vi "Build Type Tree.vi"(10 "Value":variant, 11 "Name":string) -> (3 "Type Tree":T1[](array[typedef]))   [LabVIEW 2018, in "LVClassByRef.lvlib"]
uses:
  <resource>/Framework/Providers/LVClassByRef/LVClassByRef.lvlib
  <resource>/Framework/Providers/LVClassByRef/Type Item.ctl
  <resource>/Framework/Providers/LVClassByRef/Tree Item.ctl
  <vilib>/Utility/Data Type/Type Definitions/Data Type.ctl
  <vilib>/Utility/Data Type/NI_Data Type.lvlib
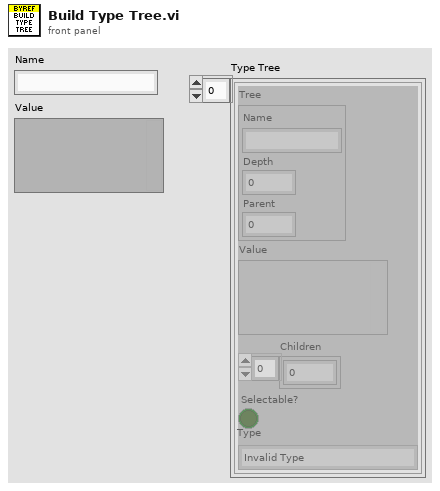
[diagram p1: front panel]
types:
  T1 = typedef "LVClassByRef.lvlib/Type Item.ctl" = cluster{"Tree":T2, "Value":variant, "Children":i32[], "Selectable?":bool, "Type":T3}
  T2 = typedef "LVClassByRef.lvlib/Tree Item.ctl" = cluster{"Name":string, "Depth":i32, "Parent":i32}
  T3 = typedef "NI_Data Type.lvlib/Data Type.ctl" = enum8{"Invalid Type", "Void", "I8", "I16", "I32", "I64", "U8", "U16", "U32", "U64", "Single Float", "Double Float", "Extended Float", "Single Complex", "Double Complex", "Extended Complex", "Enum U8", "Enum U16", "Enum U32", "Enum U64", "Single Float With Unit", "Double Float With Unit", "Extended Float With Unit", "Single Complex with Unit", "Double Complex with Unit", "Extended Complex with Unit", "Boolean", "String", "Path", "Picture", "Tag", "Array", "Cluster", "Variant", "LV Variant", "Waveform", "Timestamp", "Digital Waveform", "Digital Data", "ExpressData", "Refnum", "External Data", "VI", "Poly VI", "LabVIEW Class Instance", "Fixed Point"}
  T4 = typedef "NI_Data Type.lvlib/Refnum Type.ctl" = enum16{"NotARefnum", "UnknownRefnum", "Generic", "Datalog", "ByteStream", "Device", "Occurence", "TCPNetConnection", "Auto", "Menu", "Imaq", "Hardware", "DataSocket", "Visa", "IVI", "UDPNetConnection", "Notifier", "Queue", "Irda", "EventReg", "DotNet", "UserEvent", "Callback", "UNUSED_EMPTY_POSITION", "BlueToothNetConnection", "LVObjApp", "LVObjVI", "LVObjUnknown", "GenericClass", "UserDefinedRefnumTag", "DataValue", "RT FIFO", "TDMS File", "PythonSessionRefnum"}
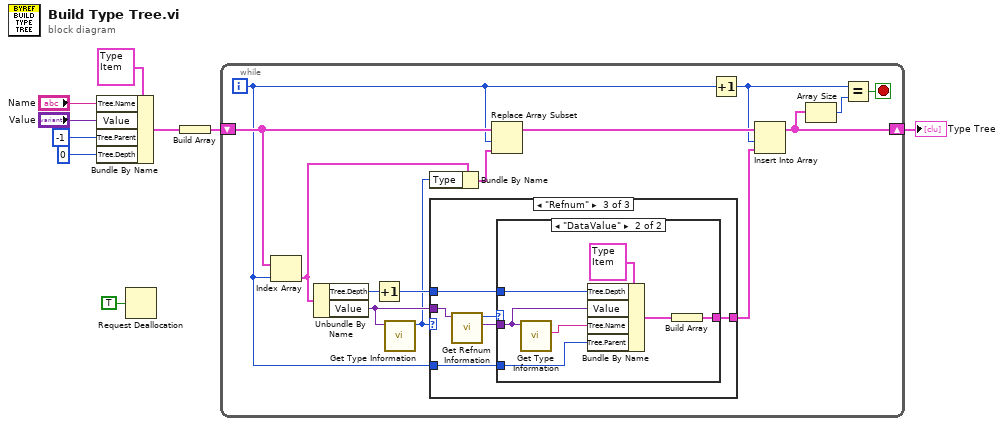
[diagram p0: block diagram]
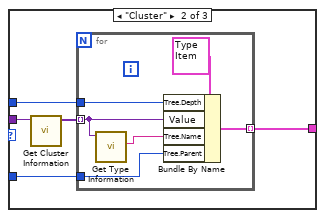
[diagram p3: hidden frame]
diagram:
  n1 = Bundle By Name(cluster=T1 {"Tree"={"Name"="", "Depth"=0, "Parent"=0}, "Value"=variant, "Children"=[], "Selectable?"=FALSE, "Type"=enum."Invalid Type"} ("Type Item"), "Tree.Name"="Name", "Value"="Value", "Tree.Parent"=-1 ("Parent Index"), "Tree.Depth"=0 ("Depth")) -> (w7:T1)
  n2 = Request Deallocation(TRUE ("flag")) -> ()
  n3 = Build Array(w7) -> (w5:T1[])
  n4 = while {
    shift-right: [w12] -> w1
    shift-left: w5 -> [w21]
    i -> [w17]
    stop <- w22 stop-if-true
    n5 = Index Array(array=w21, index=w17) -> (element=w16:T1)
    n6 = Unbundle By Name(w16) -> ("Tree.Depth"=w19:i32, "Value"=w20:variant)
    n7 = Increment(x=w19) -> (x+1=w18:i32)
    n8 = call <vilib>:"Get Type Information.vi"("Variant"=w20) -> ("Type"=w15:T3)  [unwired: 6 in, 4 out]
    n9 = Bundle By Name(cluster=w16, "Type"=w15) -> (w14:T1)
    n10 = case shown="\"Refnum\"" w15 {
      tunnel: w20 -> [_ w28 w39]
      tunnel: w17 -> [_ w27 w38]
      tunnel: [_ w25 w37] -> w11
      tunnel: w18 -> [_ w24 w36]
      frame Default {
      }
      frame "Cluster" {
        n11 = call <vilib>:"Get Cluster Information.vi"("Variant"=w28) -> ("Cluster Elements"=w26:variant[])  [unwired: 9 in, 1 out]
        n12 = for {
          tunnel: w27 -> [w31]
          tunnel: w26 -> [w32] mode=indexing
          tunnel: [w30] -> w25 mode=indexing
          tunnel: w24 -> [w29]
          n13 = call <vilib>:"Get Type Information.vi"("Variant"=w32) -> ("Name"=w33:string)  [unwired: 6 in, 4 out]
          n14 = Bundle By Name(cluster=T1 {"Tree"={"Name"="", "Depth"=0, "Parent"=0}, "Value"=variant, "Children"=[], "Selectable?"=FALSE, "Type"=enum."Invalid Type"} ("Type Item"), "Tree.Depth"=w29, "Value"=w32, "Tree.Name"=w33, "Tree.Parent"=w31) -> (w30:T1)
        }
      }
      frame "Refnum" {
        n15 = call <vilib>:"Get Refnum Information.vi"("Variant"=w39) -> ("Strict Type"=w35:variant, "Reference Type"=w40:T4)  [unwired: 7 in, 2 out]
        n16 = case shown="\"DataValue\"" w40 {
          tunnel: w38 -> [_ w46]
          tunnel: [_ w43] -> w37
          tunnel: w36 -> [_ w42]
          tunnel: w35 -> [_ w41]
          frame Default {
          }
          frame "DataValue" {
            n17 = call <vilib>:"Get Type Information.vi"("Variant"=w41) -> ("Name"=w47:string)  [unwired: 6 in, 4 out]
            n18 = Bundle By Name(cluster=T1 {"Tree"={"Name"="", "Depth"=0, "Parent"=0}, "Value"=variant, "Children"=[], "Selectable?"=FALSE, "Type"=enum."Invalid Type"} ("Type Item"), "Tree.Depth"=w42, "Value"=w41, "Tree.Name"=w47, "Tree.Parent"=w46) -> (w44:T1)
            n19 = Build Array(w44) -> (w43:T1[])
          }
        }
      }
    }
    n20 = Replace Array Subset(array=w21, new element=w14, index=w17) -> (w13:T1[])
    n21 = Increment(x=w17) -> (x+1=w10:i32)
    n22 = Insert Into Array(array=w13, index=w10, new element=w11) -> (w12:T1[])
    n23 = Array Size(array=w12) -> (size(s)=w23:i32)
    n24 = Equal?(x=w10, y=w23) -> (x = y?=w22:bool)
  }
  "Type Tree" <- w1
